vi "Load csv file to 2D table.vi"(8 "error in":errorcluster) -> (0 "error out":errorcluster, 1 "Columns":i32, 2 "Rows without header":i32, 3 "all rows":string[][](array[string]))   [LabVIEW 2024]
uses:
  <vilib>/Utility/file.llb/Read Delimited Spreadsheet (string).vi
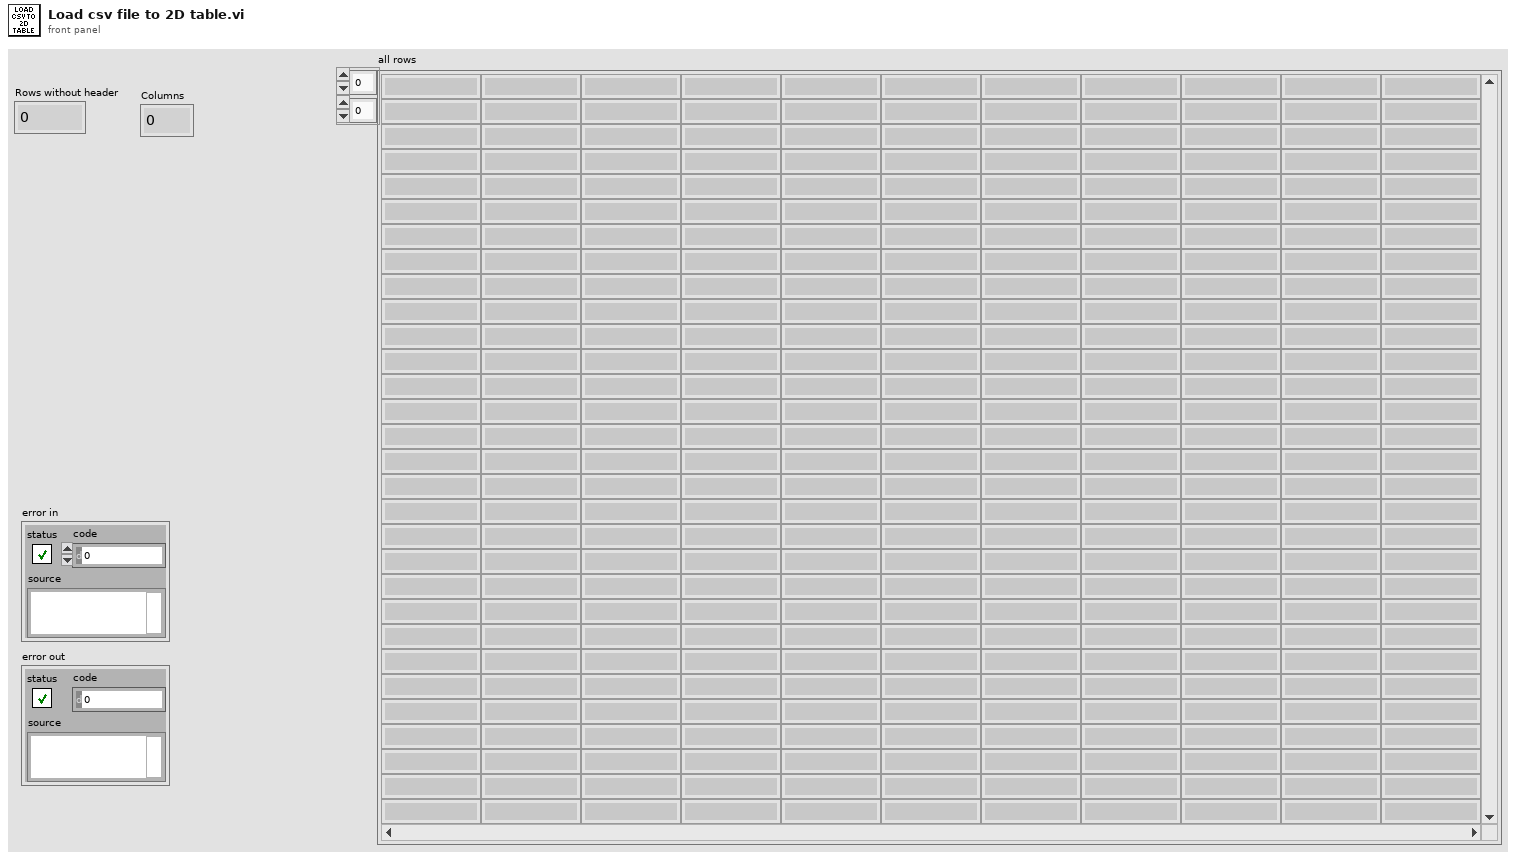
[diagram p1: front panel]
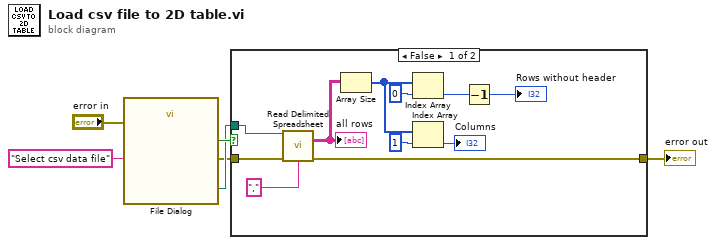
[diagram p0: block diagram]
diagram:
  n1 = call "File Dialog"("prompt"="Select csv data file", "error in"="error in") -> ("selected path"=w3:path, "cancelled"=w5:bool, "error out"=w2:errorcluster)  [unwired: 10 in, 1 out]
  n2 = case shown="False" w5 {
    tunnel: w3 -> [w16 _]
    tunnel: w2 -> [w17 w18]
    tunnel: [w15 w18] -> w1
    frame False {
      n3 = call-poly <vilib>:"Read Delimited Spreadsheet.vi"("file path (dialog if empty)"=w16, "error in (no error)"=w17, "delimiter (\\t)"="," ("delimiter (\\t)")) -> ("all rows"=w12:string[][], "error out"=w15:errorcluster)  [unwired: 7 in, 4 out]
      "all rows" <- w12
      n4 = Array Size(array=w12) -> (size(s)=w10:i32[])
      n5 = Index Array(array=w10, index=0) -> (element=w8:i32)
      n6 = Index Array(array=w10, index=1) -> (element=→"Columns":i32)
      n7 = Decrement(x=w8) -> (x-1=→"Rows without header":i32)
    }
    frame True {
    }
  }
  "error out" <- w1
